vi "Write console.vi"(8 "error in (no error)":errorcluster, 10 "console":refnum<vi>, 11 "Sink-Console in":refnum<class "Sink-Console.lvclass">) -> (0 "error out":errorcluster, 3 "Sink-Console out":refnum<class "Sink-Console.lvclass">)   [LabVIEW 2019, in "TSC Event Logger.lvlib" / "Sink-Console.lvclass"]
doc: "The console is a string control - write the reference to the console to the object.\n\n<b>Code Developed By:</b>\nTechnology Service Corporation\nBloomington, IN 47403\nwww.tsc.com/atcs\n\nDeveloper:\nDaniel Coons"
uses:
  Sink-Console.lvclass
  Sink-Console.lvclass/Sink-Console.ctl
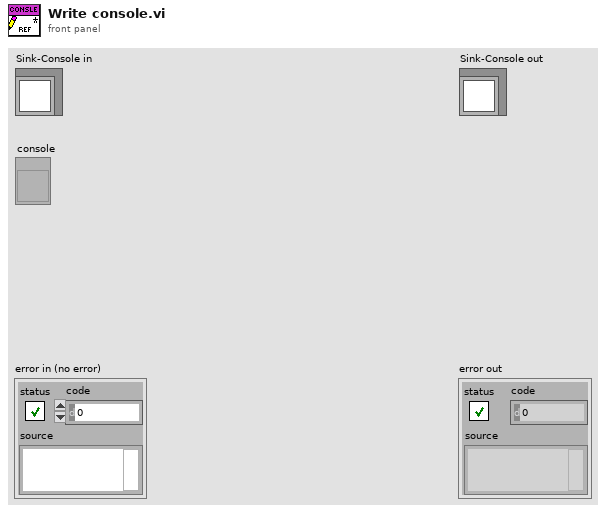
[diagram p1: front panel]
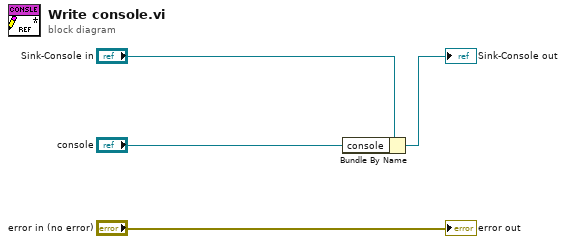
[diagram p0: block diagram]
diagram:
  n1 = Bundle By Name(cluster="Sink-Console in", "console"="console") -> (→"Sink-Console out":refnum<class "Sink-Console.lvclass">)
  "error out" <- "error in (no error)"
